vi "Create_AI_Module.vi"(8 "error in (no error)":errorcluster) -> (0 "error out":errorcluster)   [LabVIEW 2019, in "USB-87Pn.lvlib" / "USB-87Pn.lvclass"]
doc: "This VI adds a new analog input module to the USB-87Pn analog device array. This VI requires a valid address for the analog device."
uses:
  USB-87Pn.lvclass
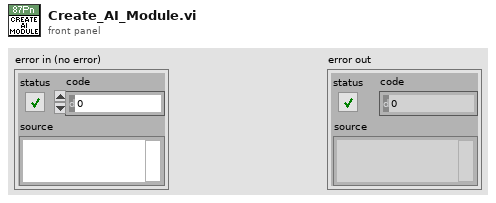
[diagram p1: front panel]
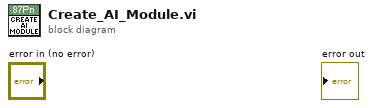
[diagram p0: block diagram]
diagram:
